vi "SetZForInte_modify_Bmode_temperature_SA Test.vi"(0 "TCP from Orchid in":refnum<k5>, 1 "timeout (ms)":dbl=40000.0 format="%.2f", 4 "RoiLaterMin":dbl format="%.2f", 5 "meas_temparature_Input":T2 {"scanRange" format="%.2f"; "temperatureC" format="%.2f"; "pulseVoltage" format="%.2f"; "roomTempC" format="%.2f"}, 9 "RoiLateralSpan":dbl format="%.2f", 11 "error in (no error)":errorcluster, 12 "meas_setting":T3={"measSetId"=6949, "measSetComments"="Orchid", "probeId"=141.0, "beamstyleIndex"=0, "txFrequencyHz"=3636400.0, "focusRangeCm"=8.0, "maxTxVoltageVolt"=100.0, "ceilTxVoltageVolt"=80.0, "profTxVoltageVolt"=62.0, "totalVoltagePt"=20, "numMeasVoltage"=12, "numTxElements"=118, "txpgWaveformStyle"=2, "numTxCycles"=4.0, "elevAperIndex"=0, "zStartDistCm"=1.5, "zMeasNum"=80, "IsTxAperModulationEn"=0, "DTxFreqIndex"=0, "VTxIndex"=0, "IsCPAEn"=0, "SysPulserSelA"=0, "TxPulseRleA"=""} {"zStartDistCm" format="%.2f"; "numTxCycles" format="%.1f"; "profTxVoltageVolt" format="%#_1g"; "ceilTxVoltageVolt" format="%.2f"; "maxTxVoltageVolt" format="%.2f"; "focusRangeCm" format="%.1f"; "txFrequencyHz" format="%.2f"}) -> (3 "Actual PRF":dbl, 6 "meas_temparature_Output":T1 {"scanRange" format="%.2f"; "txpgWaveformStyle" format="%.2f"; "temperatureC" format="%.2f"; "pulseVoltage" format="%.2f"; "roomTempC" format="%.2f"}, 10 "veri_P/F":bool, 15 "error out":errorcluster)   [LabVIEW 2016]
doc: "This VI sets the Z system transmit parameters for an intensity measurement, reads them back, and checks for errors. It first gets the initial center element delay (TxpgDelayAperA) and the system frequencies using tcpSysTxFreqFromZ.vi. It then sets the elevation aperture (using SetZElevAper.vi), channel modulation, wavestyle, frequency, focus, number of transmit elements, number of cycles, voltage, and voltage channel, in that order. It reads back the settings (using tcpReadIntenSettingsZ.vi) and checks for errors. The final trigger delay and change in delay, in microseconds, are calculated from the initial and final values of TxpgDelayAperA using:\ndelay(us) = (TxpgDelayAperA + 178.0) / 160"
uses:
  type def/measSetting.ctl
  GrobaLimitVoltage.vi
  TemperatureMeasure/Thermal_type.vi
panel:
  out "Receive array":string[](array[string])=["\r\n220 OK\r\nContainers within Hardware Control Layer\r\n\tHardwareModel\r\n\tHardwareControl\r\n\tHardwareAlgorithm\r\n\tSeq\r\n\tBeamforming\r\n\tDigitalReceiver\r\n\tEchoProcessor\r\n\tFlowProcessor\r\n\tHardwareScanConverter\r\n\tSip\r\n\tVideoInterface\r\n\tRtc\r\n\tCine\r\nScalar Parameters of Hardware Control Layer\r\nArray Parameters of Hardware Control Layer\r\ndebug\tDebug Functions\r\nquit\tExit DIOS\r\nback\tPrevious menu\r\nmain\tTop menu\r\nhelp\tAvailable commands\r\n\r\n", "\r\n220 OK\r\nContainers within Beamforming\r\n\tCommon\r\n\tBImage\r\n\tCbImage\r\n\tDImage\r\nScalar Parameters of Beamforming\r\nArray Parameters of Beamforming\r\ndebug\tDebug Functions\r\nquit\tExit DIOS\r\nback\tPrevious menu\r\nmain\tTop menu\r\nhelp\tAvailable commands\r\n\r\n", "\r\n220 OK\r\nContainers within Common\r\nScalar Parameters of Common\r\n\tBfPropagationVelCmPerSec\t154000\r\n\tDisUnit\t0.00385\r\n\tHwRcInterruptMask\t63\r\n\tHwRcTVP\t3\r\n\tHwRxAac0\t175\r\n\tHwRxAac1\t0\r\n\tHwRxbfBlankingWord\t0\r\n\tHwRxbfCmd1Word\t4232\r\n\tHwRxbfCmd2Word\t2\r\n\tHwRxbf0Cmd2Word\t3\r\n\tHwRxbfStartDelayWord\t10\r\n\tHwTiAttenuatorSelect\t0\r\n\tHwTiBitEn\t25088\r\n\tHwTiDacCtrl0\t255\r\n\tHwTiDacCtrl1\t2303\r\n\tHwTiDacCtrl2\t3327\r\n\tHwTiDacCtrl3\t511\r\n\tHwTiDacCtrl4\t2559\r\n\tHwTiDacCtrl5\t3583\r\n\tHwTiDacCtrl6\t767\r\n\tHwTiDacCtrl7\t2815\r\n\tHwTiDacCtrl8\t3839\r\n\tHwTiDacCtrl9\t2047\r\n\tHwTiDacCtrl10\t4095\r\n\tHwTiDigitalDriveCtrl\t0\r\n\tHwTiDigitalInterruptPolarity\t0\r\n\tHwTiDigitalReadCtrl\t0\r\n\tHwTiEchoBoosterCtrl\t0\r\n\tHwTiGlobalCtrl\t1\r\n\tHwTiHighVoltEn\t0\r\n\tHwTiInterruptClear\t65535\r\n\tHwTiInterruptMask\t32767\r\n\tHwTiMiscBitCtrl\t12\r\n\tHwTiProbeSelect\t2\r\n\tHwTiTXCLTransfer\t0\r\n\tHwTiVoltMultiplexer\t0\r\n\tHwTrGlobalCtrlAll\t1\r\n\tHwTrGlobalCtrl0All\t0\r\n\tHwTrDiagnosticCtrlAll\t0\r\n\tHwTrInterruptMaskAll\t1\r\n\tHwTrInterruptClearAll\t1\r\n\tHwTrRealTimeCtrlAll\t40\r\n\tHwTrTgcAacSignalCtrlAll\t0\r\n\tRxDelayRefx\t1\r\n\tRxDelayRefy\t-1\r\n\tTrPartNumber\t5928150\r\n\tBfPropagationVelFactor\t1\r\n\tDigitizingRateHz\t4e+007\r\n\tHwRxBfVectorLengthWord\t0\r\n\tIsRxVectorLengthEn\t1\r\n\tNumChannels\t192\r\n\tProbeBandwidthHz\t3.6e+006\r\n\tProbeId\t171\r\n\tProbeNumElem\t192\r\n\tProbeNumRows\t1\r\n\tProbePitchCm\t0.02\r\n\tProbeRadiusElectricalCm\t0\r\n\tProbeType\t0\r\n\tPropagationVelCmPerSec\t154000\r\n\tRxApod2dEn\t0\r\n\tRxbfAdcDelayClocks\t10\r\n\tRxbfGainShift\t0\r\n\tRxDelayYOffsetSysClk4\t0\r\n\tTxPulserMaxVolt\t50\r\nArray Parameters of Common\r\n\tHwRxbf0AdGainA\tsize=64\r\n\tHwRxbf1AdGainA\tsize=64\r\n\tHwRxbf2AdGainA\tsize=64\r\n\tHwRxbf3AdGainA\tsize=64\r\n\tHwRxbf4AdGainA\tsize=64\r\n\tHwRxbf5AdGainA\tsize=64\r\n\tHwRxbf6AdGainA\tsize=64\r\n\tHwRxbf7AdGainA\tsize=64\r\n\tHwRxbf8AdGainA\tsize=64\r\n\tHwRxbf9AdGainA\tsize=64\r\n\tHwRxbf10AdGainA\tsize=64\r\n\tHwRxbf11AdGainA\tsize=64\r\n\tHwRxAdOffsetCalA\tsize=192\r\n\tHwRxApodFilterRamA\tsize=512\r\n\tHwRxbf0DelayCalA\tsize=64\r\n\tHwRxbf1DelayCalA\tsize=64\r\n\tHwRxbf2DelayCalA\tsize=64\r\n\tHwRxbf3DelayCalA\tsize=64\r\n\tHwRxbf4DelayCalA\tsize=64\r\n\tHwRxbf5DelayCalA\tsize=64\r\n\tHwRxbf6DelayCalA\tsize=64\r\n\tHwRxbf7DelayCalA\tsize=64\r\n\tHwRxbf8DelayCalA\tsize=64\r\n\tHwRxbf9DelayCalA\tsize=64\r\n\tHwRxbf10DelayCalA\tsize=64\r\n\tHwRxbf11DelayCalA\tsize=64\r\n\tHwRxbf0DxA\tsize=64\r\n\tHwRxbf1DxA\tsize=64\r\n\tHwRxbf2DxA\tsize=64\r\n\tHwRxbf3DxA\tsize=64\r\n\tHwRxbf4DxA\tsize=64\r\n\tHwRxbf5DxA\tsize=64\r\n\tHwRxbf6DxA\tsize=64\r\n\tHwRxbf7DxA\tsize=64\r\n\tHwRxbf8DxA\tsize=64\r\n\tHwRxbf9DxA\tsize=64\r\n\tHwRxbf10DxA\tsize=64\r\n\tHwRxbf11DxA\tsize=64\r\n\tHwRxbf0DyA\tsize=64\r\n\tHwRxbf1DyA\tsize=64\r\n\tHwRxbf2DyA\tsize=64\r\n\tHwRxbf3DyA\tsize=64\r\n\tHwRxbf4DyA\tsize=64\r\n\tHwRxbf5DyA\tsize=64\r\n\tHwRxbf6DyA\tsize=64\r\n\tHwRxbf7DyA\tsize=64\r\n\tHwRxbf8DyA\tsize=64\r\n\tHwRxbf9DyA\tsize=64\r\n\tHwRxbf10DyA\tsize=64\r\n\tHwRxbf11DyA\tsize=64\r\n\tHwRxbf0DzA\tsize=128\r\n\tHwRxbf1DzA\tsize=128\r\n\tHwRxbf2DzA\tsize=128\r\n\tHwRxbf3DzA\tsize=128\r\n\tHwRxbf4DzA\tsize=128\r\n\tHwRxbf5DzA\tsize=128\r\n\tHwRxbf6DzA\tsize=128\r\n\tHwRxbf7DzA\tsize=128\r\n\tHwRxbf8DzA\tsize=128\r\n\tHwRxbf9DzA\tsize=128\r\n\tHwRxbf10DzA\tsize=128\r\n\tHwRxbf11DzA\tsize=128\r\n\tHwRxbf0PosInApodWinA\tsize=64\r\n\tHwRxbf1PosInApodWinA\tsize=64\r\n\tHwRxbf2PosInApodWinA\tsize=64\r\n\tHwRxbf3PosInApodWinA\tsize=64\r\n\tHwRxbf4PosInApodWinA\tsize=64\r\n\tHwRxbf5PosInApodWinA\tsize=64\r\n\tHwRxbf6PosInApodWinA\tsize=64\r\n\tHwRxbf7PosInApodWinA\tsize=64\r\n\tHwRxbf8PosInApodWinA\tsize=64\r\n\tHwRxbf9PosInApodWinA\tsize=64\r\n\tHwRxbf10PosInApodWinA\tsize=64\r\n\tHwRxbf11PosInApodWinA\tsize=64\r\n\tHwRxMuxSelectLutA\tsize=512\r\n\tHwRxRamOffsetA\tsize=12\r\n\tHwTxDacA\tsize=2\r\n\tHwTxpgDelayAperA\tsize=393216\r\n\tNumBitsPerCycleA\tsize=49\r\n\tNumCyclesPerPassA\tsize=49\r\n\tNumWordsPerPassA\tsize=49\r\n\tRxAdGainA\tsize=256\r\n\tRxDelayCalA\tsize=768\r\n\tRxDxA\tsize=256\r\n\tRxDyA\tsize=256\r\n\tRxDzA\tsize=256\r\n\tRxMuxSelectLutPtrA\tsize=512\r\n\tRxPosInApodWinA\tsize=768\r\n\tTxDelayCalA\tsize=192\r\n\tTxpgWaveformHoutA\tsize=15680\r\n\tTxpgWaveformLoutA\tsize=15680\r\n\tYIndexTableA\tsize=256\r\n\tZIndexTableA\tsize=256\r\n\tInsertedProbeIdA\tsize=6\r\n\tPulseVoltageA\tsize=2\r\n\tRxApodFactorA\tsize=4\r\n\tRxApodSelA\tsize=4\r\n\tSysTxFreqHzA\tsize=49\r\ndebug\tDebug Functions\r\nquit\tExit DIOS\r\nback\tPrevious menu\r\nmain\tTop menu\r\nhelp\tAvailable commands\r\n\r\n", "220 OK\r\n", "250 20\r\n"]
  out "error out 2":errorcluster
  out "Pass_count":i16
  out "All_param_veri":bool[](array[boolean])
  in  "volt channel":i8
  # "Program constants"
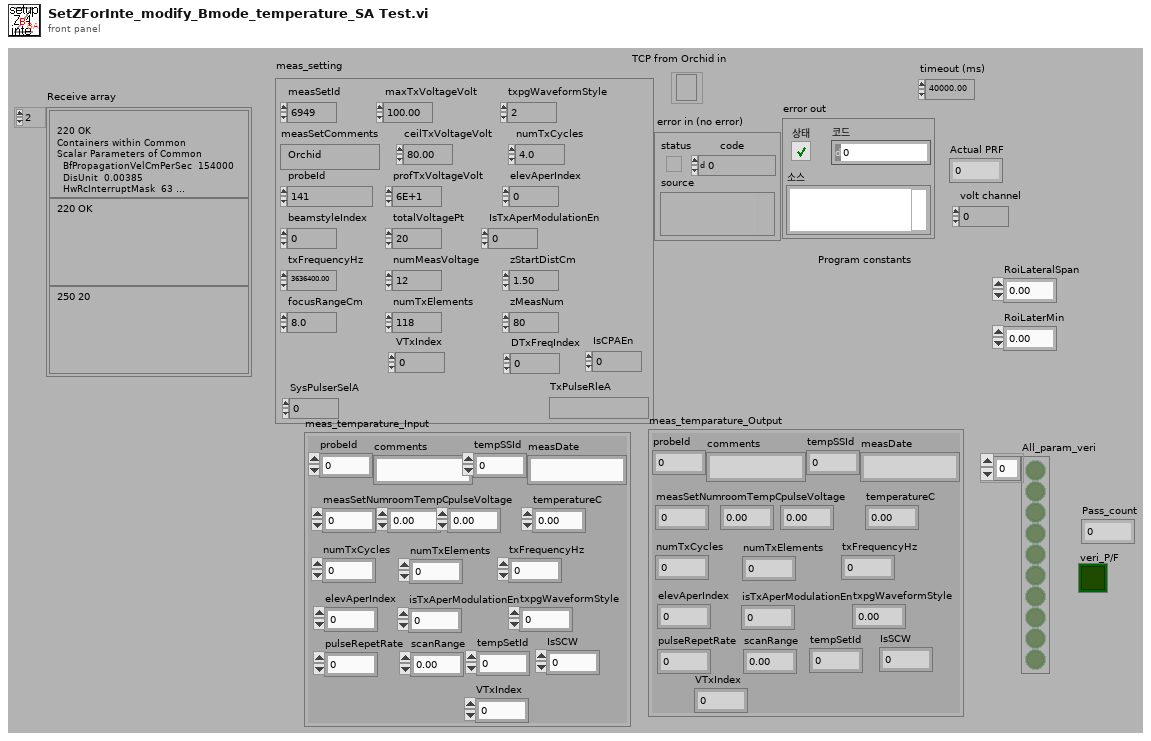
[diagram p1: front panel]
types:
  T1 = cluster{"probeId":sgl, "comments":string, "tempSSId":i16, "measDate":string, "measSetNum":i16, "roomTempC":sgl, "pulseVoltage":dbl, "temperatureC":ext, "numTxCycles":dbl, "numTxElements":i16, "txFrequencyHz":i32, "elevAperIndex":i16, "isTxAperModulationEn":i16, "txpgWaveformStyle":sgl, "pulseRepetRate":i32, "scanRange":dbl, "tempSetId":i16, "IsSCW":i16, "VTxIndex":i32}
  T2 = cluster{"probeId":sgl, "comments":string, "tempSSId":i16, "measDate":string, "measSetNum":i16, "roomTempC":sgl, "pulseVoltage":dbl, "temperatureC":ext, "numTxCycles":dbl, "numTxElements":i16, "txFrequencyHz":i32, "elevAperIndex":i16, "isTxAperModulationEn":i16, "txpgWaveformStyle":i16, "pulseRepetRate":dbl, "scanRange":dbl, "tempSetId":i16, "IsSCW":i16, "VTxIndex":i16}
  T3 = typedef "measSetting.ctl" = cluster{"measSetId":i32, "measSetComments":string, "probeId":sgl, "beamstyleIndex":i16, "txFrequencyHz":sgl, "focusRangeCm":sgl, "maxTxVoltageVolt":sgl, "ceilTxVoltageVolt":sgl, "profTxVoltageVolt":dbl, "totalVoltagePt":i8, "numMeasVoltage":i8, "numTxElements":i16, "txpgWaveformStyle":i8, "numTxCycles":sgl, "elevAperIndex":i8, "zStartDistCm":sgl, "zMeasNum":i8, "IsTxAperModulationEn":i8, "DTxFreqIndex":i16, "VTxIndex":i8, "IsCPAEn":i16, "SysPulserSelA":i16, "TxPulseRleA":string}
  T4 = cluster{"numTxCycles":dbl, "numTxElements":i16, "txFrequencyIndex":i32, "isTxAperModulationEn":i16, "txpgWaveformStyle":i16, "pulseRepetRate":dbl, "RoiLateralSpan":dbl, "RoiLateralMin":dbl}
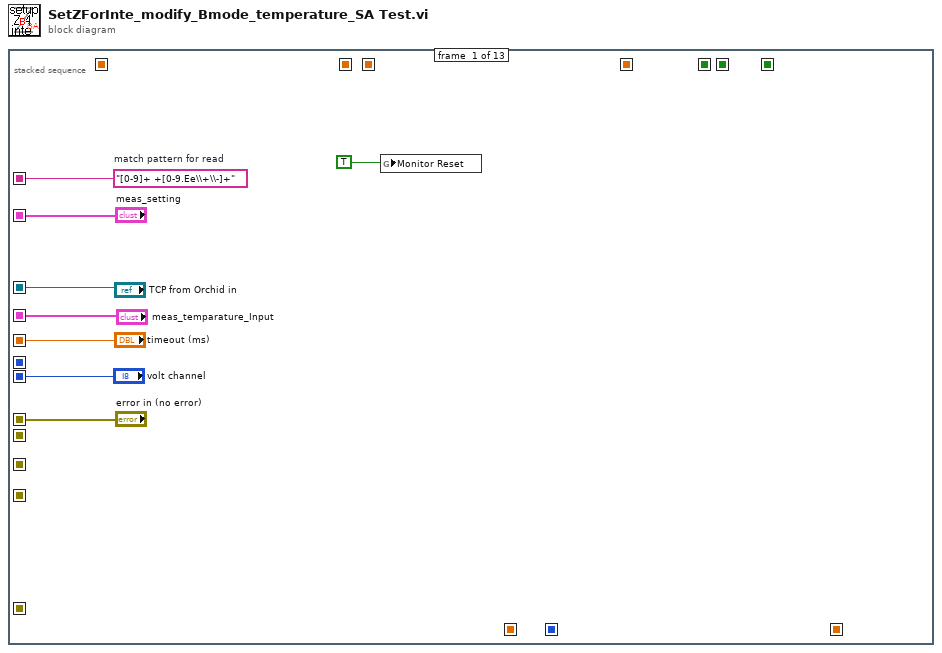
[diagram p0: block diagram]
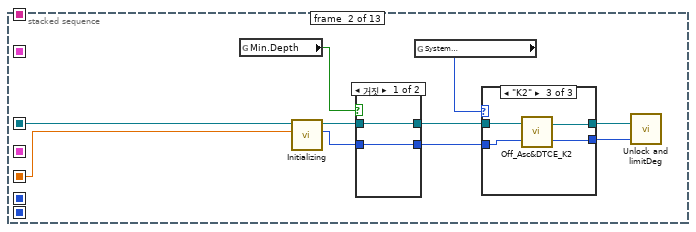
[diagram p2: hidden frame]
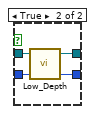
[diagram p3: hidden frame]
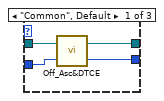
[diagram p4: hidden frame]
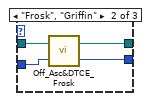
[diagram p5: hidden frame]
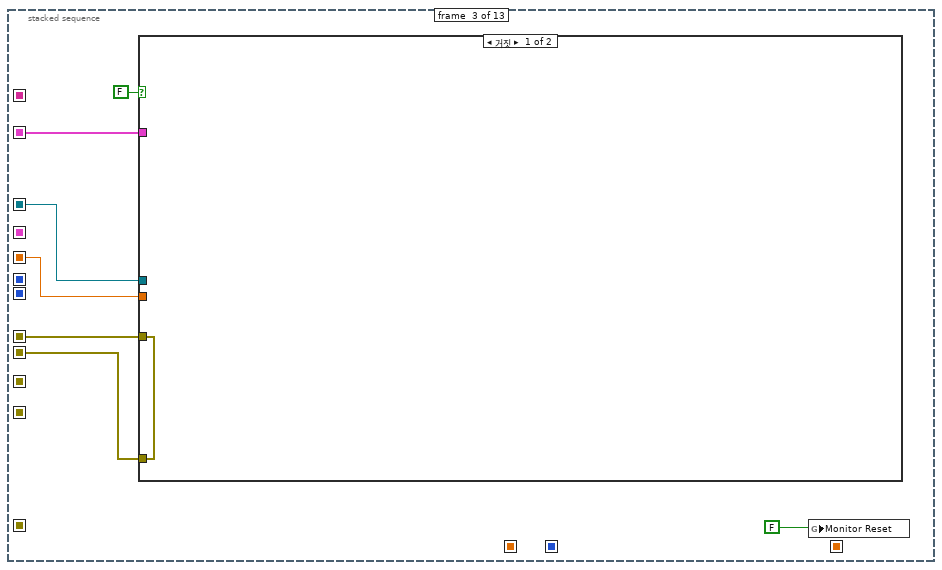
[diagram p6: hidden frame]
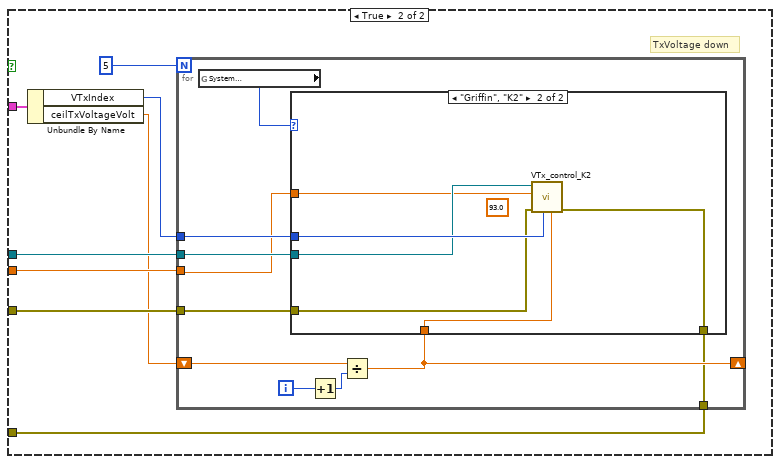
[diagram p7: hidden frame]
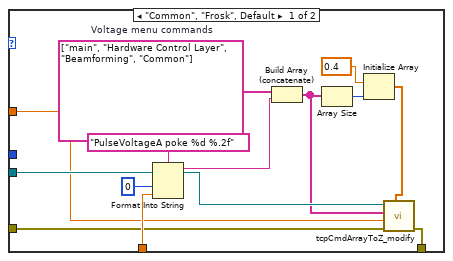
[diagram p8: hidden frame]
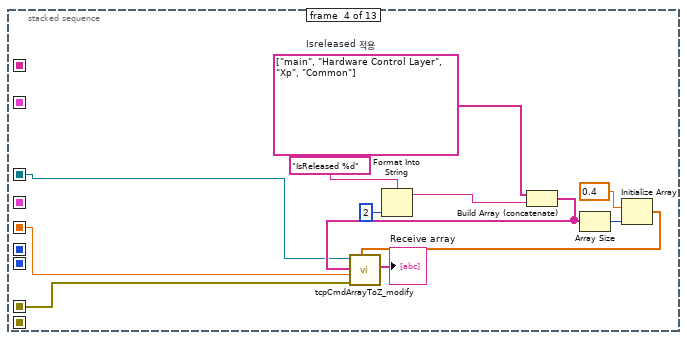
[diagram p9: hidden frame]
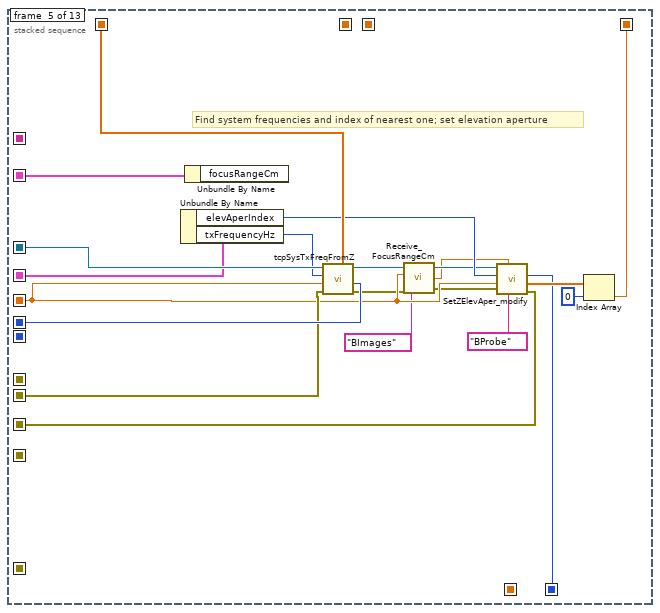
[diagram p10: hidden frame]
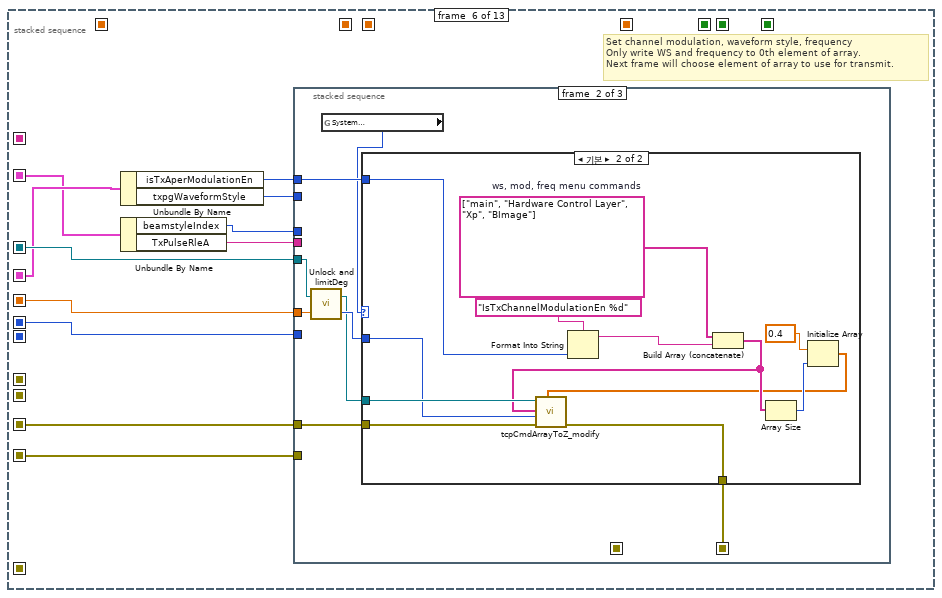
[diagram p11: hidden frame]
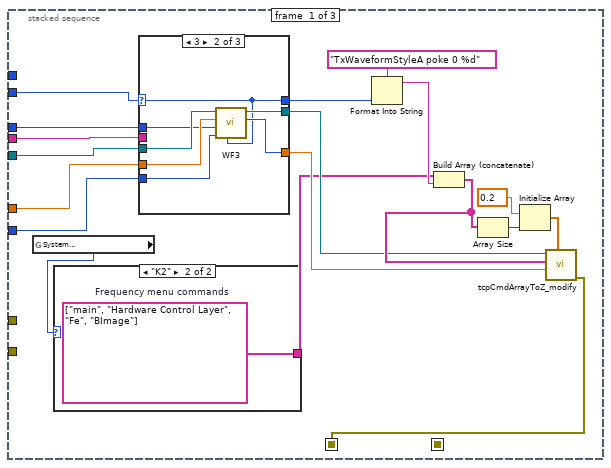
[diagram p12: hidden frame]
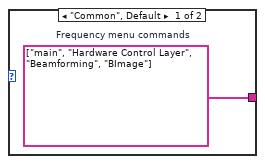
[diagram p13: hidden frame]
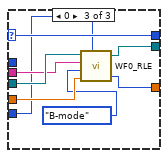
[diagram p15: hidden frame]
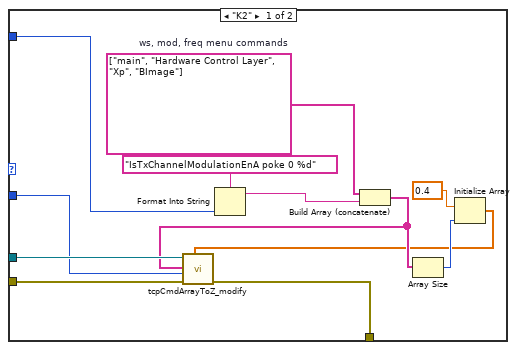
[diagram p16: hidden frame]
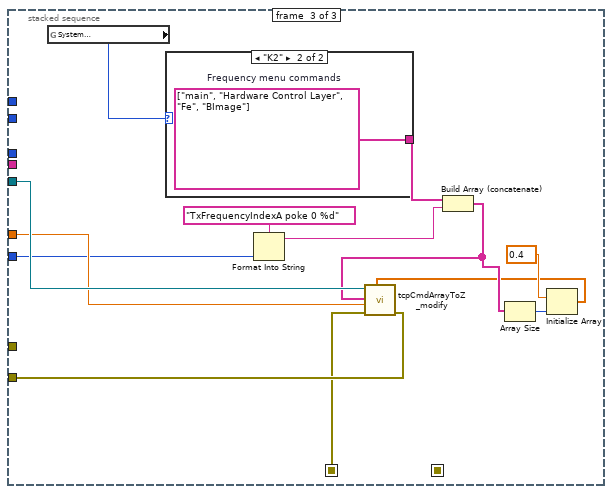
[diagram p17: hidden frame]
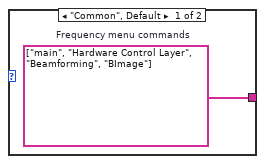
[diagram p18: hidden frame]
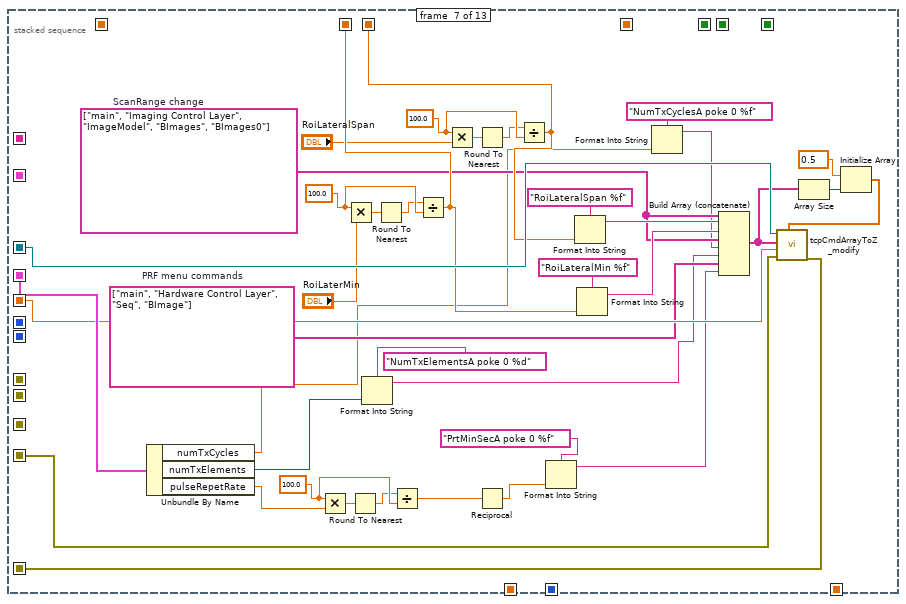
[diagram p19: hidden frame]
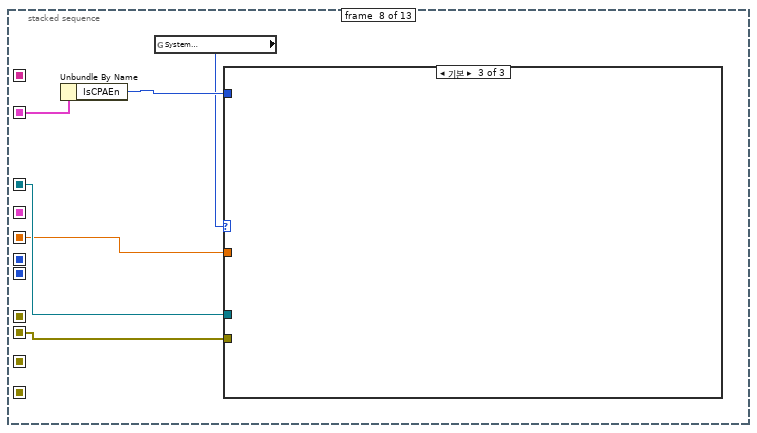
[diagram p20: hidden frame]
diagram:
  n1 = stacked-sequence {
    seq-local: ["meas_temparature_Input" _ _ _ _ _ _ _ _ _ _ _ _] -> [_ _ _ _ w113 w120 w249 _ _ w336 w359 _ _]
    seq-local: ["TCP from Orchid in" _ _ _ _ _ _ _ _ _ _ _ _] -> [_ w18 w41 w84 w114 w125 w247 w255 w281 w335 w352 w400 w414]
    seq-local: ["timeout (ms)" _ _ _ _ _ _ _ _ _ _ _ _] -> [_ w17 w40 w82 w97 w124 w246 w254 w280 w334 w351 w399 w413]
    seq-local: [_ _ _ _ w112 _ _ _ _ _ _ _ _] -> [_ _ _ _ _ w121 _ _ _ w340 _ _ _]
    seq-local: [_ _ _ _ w104 _ _ _ _ _ _ _ _] -> [_ _ _ _ _ w122 _ _ _ _ _ _ _]
    seq-local: [_ _ _ _ w111 _ _ _ _ _ _ _ _] -> [_ _ _ _ _ _ _ _ _ _ _ _ _]
    seq-local: ["volt channel" _ _ _ _ _ _ _ _ _ _ _ _] -> [_ _ _ _ _ _ _ _ _ _ _ _ _]
    seq-local: ["error in (no error)" _ _ _ _ _ _ _ _ _ _ _ _] -> [_ _ w39 w83 _ _ _ _ _ _ _ _ _]
    seq-local: [w5 _ _ _ _ _ _ _ _ _ _ _ _] -> [_ _ _ _ _ _ _ _ _ _ _ _ _]
    seq-local: [_ _ w38 _ _ _ _ _ _ _ _ _ _] -> [_ _ _ _ w109 _ _ w252 w279 _ _ _ _]
    seq-local: [_ _ _ _ _ w123 _ _ _ _ _ _ _] -> [_ _ _ _ _ _ w248 _ _ _ _ _ _]
    seq-local: [_ _ _ _ _ _ w245 _ _ _ _ _ _] -> [_ _ _ _ _ _ _ _ _ _ w349 _ _]
    seq-local: ["meas_setting" _ _ _ _ _ _ _ _ _ _ _ _] -> [_ _ w43 _ w102 w119 _ w253 _ w316 w354 _ _]
    seq-local: [_ _ _ _ _ _ w243 _ _ _ _ _ _] -> [_ _ _ _ _ _ _ _ _ w338 _ _ _]
    seq-local: [_ _ _ _ _ _ w244 _ _ _ _ _ _] -> [_ _ _ _ _ _ _ _ _ w339 _ _ _]
    seq-local: [_ _ _ _ _ _ _ _ _ _ w348 _ _] -> [_ _ _ _ _ _ _ _ _ _ _ _ _]
    seq-local: [_ _ _ _ _ _ _ _ _ w337 _ _ _] -> [_ _ _ _ _ _ _ _ _ _ _ w398 _]
    seq-local: [_ _ _ _ _ _ _ _ _ _ w346 _ _] -> [_ _ _ _ _ _ _ _ _ _ _ w397 _]
    seq-local: [_ _ _ _ w103 _ _ _ _ _ _ _ _] -> [_ _ _ _ _ _ _ _ _ _ _ _ _]
    seq-local: [_ _ _ _ w101 _ _ _ _ _ _ _ _] -> [_ _ _ _ _ _ _ _ _ _ _ _ _]
    seq-local: [_ _ _ _ _ _ _ _ _ w312 _ _ _] -> [_ _ _ _ _ _ _ _ _ _ _ w395 _]
    seq-local: [_ _ _ _ _ _ _ _ w278 _ _ _ _] -> [_ _ _ _ _ _ _ _ _ w310 _ _ _]
    frame #0 {
      w5 = "[0-9]+ +[0-9.Ee\\+\\-]+"  # match pattern for read
      n2 = global write "GrobaLimitVoltage.vi" "Monitor Reset"(TRUE) -> ()
    }
    frame #1 {
      n3 = global read "Thermal_type.vi" "Min.Depth"() -> (w9:bool)
      n4 = call "Initializing.vi"("Timeout (ms)"=w17, "connection ID in"=w18) -> ("Timeout (ms) 2"=w12:i32, "connection ID in 2"=w13:refnum<k5>)  [unwired: 8 in]
      n5 = case shown="거짓" w9 {
        tunnel: w13 -> [w20 w24]
        tunnel: w12 -> [w19 w23]
        tunnel: [w20 w22] -> w11
        tunnel: [w19 w21] -> w10
        frame False {
        }
        frame True {
          n6 = call "Low_Depth.vi"("Timeout (ms)"=w23, "connection ID in"=w24) -> ("Timeout (ms) 2"=w21:i32, "connection ID out"=w22:refnum<k5>)  [unwired: 2 in]
        }
      }
      n7 = global read "Thermal_type.vi" "System \nSelection"() -> (w16:enum32{"Common", "Frosk", "Griffin", "K2"})
      n8 = case shown="\"K2\"" w16 {
        tunnel: [w28 w32 w34] -> w15
        tunnel: [w27 w31 w33] -> w14
        tunnel: w11 -> [w26 w30 w36]
        tunnel: w10 -> [w25 w29 w35]
        frame "Common", Default {
          n9 = call "Off_Asc&DTCE.vi"("Timeout (ms)"=w25, "connection ID in"=w26) -> ("Timeout (ms) 2"=w27:i32, "connection ID out"=w28:refnum<k5>)
        }
        frame "Frosk", "Griffin" {
          n10 = call "Off_Asc&DTCE_Frosk.vi"("Timeout (ms)"=w29, "connection ID in"=w30) -> ("Timeout (ms) 2"=w31:i32, "connection ID out"=w32:refnum<k5>)
        }
        frame "K2" {
          n11 = call "Off_Asc&DTCE_K2.vi"("Timeout (ms)"=w35, "connection ID in"=w36) -> ("Timeout (ms) 2"=w33:i32, "connection ID out"=w34:refnum<k5>)
        }
      }
      n12 = call "Unlock and limitDeg.vi"("Timeout (ms)"=w14, "connection ID in"=w15) -> ()  [unwired: 2 out]
    }
    frame #2 {
      n13 = case shown="거짓" FALSE {
        tunnel: w43 -> [_ w52]
        tunnel: w41 -> [_ w49]
        tunnel: w40 -> [_ w48]
        tunnel: w39 -> [w44 w47]
        tunnel: [w44 w46] -> w38
        frame False {
        }
        frame True {
          # "TxVoltage down"
          n14 = Unbundle By Name(w52) -> ("VTxIndex"=w50:i8, "ceilTxVoltageVolt"=w45:sgl)
          n15 = for {
            N: 5 -> [_]
            tunnel: w49 -> [w62]
            shift-right: [w56] -> _
            shift-left: w45 -> [w58]
            tunnel: w50 -> [w61]
            tunnel: [w55] -> w46
            tunnel: w48 -> [w54]
            tunnel: w47 -> [w53]
            i -> [w57]
            n16 = global read "Thermal_type.vi" "System \nSelection"() -> (w60:enum32{"Common", "Frosk", "Griffin", "K2"})
            n17 = Increment(x=w57) -> (x+1=w59:i32)
            n18 = Divide(x=w58, y=w59) -> (x/y=w56:sgl)
            n19 = case shown="\"Griffin\", \"K2\"" w60 {
              tunnel: w62 -> [w75 w80]
              tunnel: w61 -> [_ w81]
              tunnel: w56 -> [w66 w79]
              tunnel: [w65 w78] -> w55
              tunnel: w54 -> [w63 w77]
              tunnel: w53 -> [w64 w76]
              frame "Common", "Frosk", Default {
                w73 = string[] ["main", "Hardware Control Layer", "Beamforming", "Common"]  # Voltage menu commands
                n20 = Format Into String(format string="PulseVoltageA poke %d %.2f" ("Format String"), i8 0 ("입력 1"), w66) -> (resulting string=w72:string)  [unwired: 2 in, 1 out]
                n21 = Build Array (concatenate)(w73, w72) -> (w68:string[])
                n22 = Array Size(array=w68) -> (size(s)=w71:i32)
                n23 = Initialize Array(0.4 ("element"), w71) -> (w69:dbl[])
                n24 = call "tcpCmdArrayToZ_modify.vi"("Delay (sec)"=w69, "error in (no error)"=w64, "Timeout (ms)"=w63, "Command array"=w68, "connection ID in"=w75) -> ("error out"=w65:errorcluster)  [unwired: 2 in, 4 out]
              }
              frame "Griffin", "K2" {
                (unwired) 93.0 ("VTx1_voltage")
                n25 = call "VTx_control_K2.vi"("VTx_Voltage"=w79, "VTxIndex_In"=w81, "error in (no error)"=w76, "Timeout (ms)"=w77, "connection ID in"=w80) -> ("error out"=w78:errorcluster)  [unwired: 5 in, 1 out]
              }
            }
          }
        }
      }
      n26 = global write "GrobaLimitVoltage.vi" "Monitor Reset"(FALSE) -> ()
    }
    frame #3 {
      w87 = string[] ["main", "Hardware Control Layer", "Xp", "Common"]  # Isreleased 적용
      n27 = Format Into String(format string="IsReleased %d" ("Format String"), i16 2 ("입력 1")) -> (resulting string=w92:string)  [unwired: 2 in, 1 out]
      n28 = Build Array (concatenate)(w87, w92) -> (w89:string[])
      n29 = Array Size(array=w89) -> (size(s)=w91:i32)
      n30 = Initialize Array(0.4 ("element"), w91) -> (w88:dbl[])
      n31 = call "tcpCmdArrayToZ_modify.vi"("Delay (sec)"=w88, "error in (no error)"=w83, "Timeout (ms)"=w82, "Command array"=w89, "connection ID in"=w84) -> ("Receive array"=→"Receive array":string[])  [unwired: 2 in, 4 out]
    }
    frame #4 {
      # "Find system frequencies and index of nearest one; set elevation aperture"
      n32 = Unbundle By Name(w113) -> ("elevAperIndex"=w105:i16, "txFrequencyHz"=w110:i32)
      n33 = Unbundle By Name(w102) -> ()  [unwired: 1 out]
      n34 = call "tcpSysTxFreqFromZ.vi"("error in (no error)"=w109, "timeout (ms)"=w97, "txFrequencyHz in"=w110, "connection ID in"=w114) -> ("error out"=w95:errorcluster, "TxFreqIndex"=w112:i8, "connection ID out"=w100:refnum<k5>, "SysTxFreqHzA"=w111:sgl[])  [unwired: 3 in, 1 out]
      n35 = call "Receive_FocusRangeCm.vi"("error in (no error)"=w95, "Image mode"="BImages", "Timeout (ms)"=w97, "connection ID in"=w100) -> ("error out"=w94:errorcluster, "FocusRangeCm"=w98:dbl, "connection ID out"=w99:refnum<k5>)
      n36 = call "SetZElevAper_modify.vi"("Mode"="BProbe", "focusRangeCm"=w98, "error in (no error)"=w94, "timeout (ms)"=w97, "elevAperIndex"=w105, "connection ID in"=w99) -> ("error out"=w104:errorcluster, "SwitchDepth"=w107:sgl[], "probeNumElevAper"=w103:i32)  [unwired: 2 in, 1 out]
      n37 = Index Array(array=w107, index=0 ("인덱스")) -> (element=w101:sgl)
    }
    frame #5 {
      # "Set channel modulation, waveform style, frequency\nOnly write WS and frequency to 0th element of array.\nNext frame will choose element of array to use for transmit."
      n38 = Unbundle By Name(w120) -> ("isTxAperModulationEn"=w118:i16, "txpgWaveformStyle"=w117:i16)
      n39 = Unbundle By Name(w119) -> ("beamstyleIndex"=w116:i16, "TxPulseRleA"=w115:string)
      n40 = stacked-sequence {
        seq-local: [w128 _ _] -> [_ _ w196]
        seq-local: [_ w169 _] -> [_ _ _]
        tunnel: w125 -> [w138 w165 w208]
        tunnel: w124 -> [w137 w164 w207]
        tunnel: [_ _ w206] -> w123
        tunnel: w122 -> [_ w170 _]
        tunnel: w121 -> [w136 _ w204]
        tunnel: w118 -> [_ w171 _]
        tunnel: w117 -> [w127 _ _]
        tunnel: w116 -> [w135 _ _]
        tunnel: w115 -> [w126 _ _]
        frame #0 {
          n41 = global read "Thermal_type.vi" "System \nSelection"() -> (w129:enum32{"Common", "Frosk", "Griffin", "K2"})
          n42 = case shown="\"K2\"" w129 {
            tunnel: [w144 w145] -> w130
            frame "Common", Default {
              w144 = string[] ["main", "Hardware Control Layer", "Beamforming", "BImage"]  # Frequency menu commands
            }
            frame "K2" {
              w145 = string[] ["main", "Hardware Control Layer", "Fe", "BImage"]  # Frequency menu commands
            }
          }
          n43 = case shown="3" w127 {
            selector: w127 -> [w146 w149 w160]
            tunnel: w138 -> [w148 w155 w163]
            tunnel: [w148 w154 w159] -> w133
            tunnel: [w147 w153 w158] -> w132
            tunnel: w137 -> [w147 w152 w161]
            tunnel: w135 -> [_ w151 _]
            tunnel: w136 -> [_ w150 w156]
            tunnel: [w146 w149 w160] -> w134
            tunnel: w126 -> [_ _ w162]
            frame Default {
            }
            frame 3 {
              n44 = call "WF3.vi"("TxWaveformStyle"=w149, "TxFreqIndex"=w150, "BeamStyleIndex"=w151, "Timeout (ms)"=w152, "connection ID in"=w155) -> ("Timeout (ms) out"=w153:i32, "connection ID out"=w154:refnum<k5>)  [unwired: 5 in]
            }
            frame 0 {
              n45 = call "WF0_RLE.vi"("connection ID in"=w163, "TxPulseRleA"=w162, "Mode control"=enum32{"D-mode", "B-mode"}."B-mode", "Timeout (ms)"=w161, "TxFrequencyIndex"=w156) -> ("connection ID out"=w159:refnum<k5>, "Timeout (ms) out"=w158:i32)  [unwired: 1 in]
            }
          }
          n46 = Format Into String(format string="TxWaveformStyleA poke 0 %d" ("Format String"), w134) -> (resulting string=w131:string)  [unwired: 2 in, 1 out]
          n47 = Build Array (concatenate)(w130, w131) -> (w140:string[])
          n48 = Array Size(array=w140) -> (size(s)=w142:i32)
          n49 = Initialize Array(0.2 ("element"), w142) -> (w139:dbl[])
          n50 = call "tcpCmdArrayToZ_modify.vi"("Delay (sec)"=w139, "Timeout (ms)"=w132, "Command array"=w140, "connection ID in"=w133) -> ("error out"=w128:errorcluster)  [unwired: 3 in, 4 out]
        }
        frame #1 {
          n51 = call "Unlock and limitDeg.vi"("Timeout (ms)"=w164, "connection ID in"=w165) -> ("Timeout (ms) 2"=w167:i32, "connection ID out"=w166:refnum<k5>)
          n52 = global read "Thermal_type.vi" "System \nSelection"() -> (w168:enum32{"Common", "Frosk", "Griffin", "K2"})
          n53 = case shown="기본" w168 {
            tunnel: w166 -> [w183 w195]
            tunnel: w167 -> [w182 w194]
            tunnel: w171 -> [w175 w187]
            tunnel: w170 -> [w173 w185]
            tunnel: [w172 w184] -> w169
            frame "K2" {
              w174 = string[] ["main", "Hardware Control Layer", "Xp", "BImage"]  # ws, mod, freq menu commands
              n54 = Format Into String(format string="IsTxChannelModulationEnA poke 0 %d" ("Format String"), w175) -> (resulting string=w180:string)  [unwired: 2 in, 1 out]
              n55 = Build Array (concatenate)(w174, w180) -> (w177:string[])
              n56 = Array Size(array=w177) -> (size(s)=w179:i32)
              n57 = Initialize Array(0.4 ("element"), w179) -> (w176:dbl[])
              n58 = call "tcpCmdArrayToZ_modify.vi"("Delay (sec)"=w176, "error in (no error)"=w173, "Timeout (ms)"=w182, "Command array"=w177, "connection ID in"=w183) -> ("error out"=w172:errorcluster)  [unwired: 2 in, 4 out]
            }
            frame Default {
              w186 = string[] ["main", "Hardware Control Layer", "Xp", "BImage"]  # ws, mod, freq menu commands
              n59 = Format Into String(format string="IsTxChannelModulationEn %d" ("Format String"), w187) -> (resulting string=w192:string)  [unwired: 2 in, 1 out]
              n60 = Build Array (concatenate)(w186, w192) -> (w189:string[])
              n61 = Array Size(array=w189) -> (size(s)=w191:i32)
              n62 = Initialize Array(0.4 ("element"), w191) -> (w188:dbl[])
              n63 = call "tcpCmdArrayToZ_modify.vi"("Delay (sec)"=w188, "error in (no error)"=w185, "Timeout (ms)"=w194, "Command array"=w189, "connection ID in"=w195) -> ("error out"=w184:errorcluster)  [unwired: 2 in, 4 out]
            }
          }
        }
        frame #2 {
          n64 = global read "Thermal_type.vi" "System \nSelection"() -> (w198:enum32{"Common", "Frosk", "Griffin", "K2"})
          n65 = case shown="\"K2\"" w198 {
            tunnel: [w209 w210] -> w197
            frame "Common", Default {
              w209 = string[] ["main", "Hardware Control Layer", "Beamforming", "BImage"]  # Frequency menu commands
            }
            frame "K2" {
              w210 = string[] ["main", "Hardware Control Layer", "Fe", "BImage"]  # Frequency menu commands
            }
          }
          n66 = Format Into String(format string="TxFrequencyIndexA poke 0 %d" ("Format String"), w204) -> (resulting string=w203:string)  [unwired: 2 in, 1 out]
          n67 = Build Array (concatenate)(w197, w203) -> (w200:string[])
          n68 = Array Size(array=w200) -> (size(s)=w202:i32)
          n69 = Initialize Array(0.4 ("element"), w202) -> (w199:dbl[])
          n70 = call "tcpCmdArrayToZ_modify.vi"("Delay (sec)"=w199, "error in (no error)"=w196, "Timeout (ms)"=w207, "Command array"=w200, "connection ID in"=w208) -> ("error out"=w206:errorcluster)  [unwired: 2 in, 4 out]
        }
      }
    }
    frame #6 {
      w219 = 100.0
      w223 = 100.0
      w227 = 100.0
      w232 = string[] ["main", "Imaging Control Layer", "ImageModel", "BImages", "BImages0"]  # ScanRange change
      w234 = string[] ["main", "Hardware Control Layer", "Seq", "BImage"]  # PRF menu commands
      n71 = Unbundle By Name(w249) -> ("numTxCycles"=w229:dbl, "numTxElements"=w236:i16, "pulseRepetRate"=w217:dbl)
      n72 = Multiply(x=w219, y=w217) -> (x*y=w220:dbl)
      n73 = Multiply(x=w223, y="RoiLaterMin") -> (x*y=w224:dbl)
      n74 = Round To Nearest(number=w220) -> (nearest integer value=w218:dbl)
      n75 = Format Into String(format string="NumTxElementsA poke 0 %d" ("Format String"), w236) -> (resulting string=w233:string)  [unwired: 2 in, 1 out]
      n76 = Round To Nearest(number=w224) -> (nearest integer value=w222:dbl)
      n77 = Divide(x=w218, y=w219) -> (x/y=w212:dbl)
      n78 = Divide(x=w222, y=w223) -> (x/y=w243:dbl)
      n79 = Multiply(x=w227, y="RoiLateralSpan") -> (x*y=w228:dbl)
      n80 = Round To Nearest(number=w228) -> (nearest integer value=w226:dbl)
      n81 = Reciprocal(x=w212) -> (1/x=w211:dbl)
      n82 = Divide(x=w226, y=w227) -> (x/y=w244:dbl)
      n83 = Format Into String(format string="PrtMinSecA poke 0 %f", w211) -> (resulting string=w235:string)  [unwired: 2 in, 1 out]
      n84 = Format Into String(format string="RoiLateralSpan %f", w244) -> (resulting string=w239:string)  [unwired: 2 in, 1 out]
      n85 = Format Into String(format string="RoiLateralMin %f", w243) -> (resulting string=w238:string)  [unwired: 2 in, 1 out]
      n86 = Format Into String(format string="NumTxCyclesA poke 0 %f" ("Format String"), w229) -> (resulting string=w230:string)  [unwired: 2 in, 1 out]
      n87 = Build Array (concatenate)(w232, w239, w238, w232, w230, w233, w234, w235) -> (w214:string[])
      n88 = Array Size(array=w214) -> (size(s)=w216:i32)
      n89 = Initialize Array(0.5 ("element"), w216) -> (w213:dbl[])
      n90 = call "tcpCmdArrayToZ_modify.vi"("Delay (sec)"=w213, "error in (no error)"=w248, "Timeout (ms)"=w246, "Command array"=w214, "connection ID in"=w247) -> ("error out"=w245:errorcluster)  [unwired: 2 in, 4 out]
    }
    frame #7 {
      n91 = Unbundle By Name(w253) -> ("IsCPAEn"=w251:i16)
      n92 = global read "Thermal_type.vi" "System \nSelection"() -> (w250:enum32{"Common", "Frosk", "Griffin", "K2"})
      n93 = case shown="기본" w250 {
        tunnel: w255 -> [w266 w277 _]
        tunnel: w254 -> [w265 w276 _]
        tunnel: w251 -> [w258 w269 _]
        tunnel: w252 -> [w256 w267 _]
        frame "K2" {
          w257 = string[] ["main", "Hardware Control Layer", "Fe", "BImage"]  # ws, mod, freq menu commands
          n94 = Format Into String(format string="IsCPAEn %d" ("Format String"), w258) -> (resulting string=w263:string)  [unwired: 2 in, 1 out]
          n95 = Build Array (concatenate)(w257, w263) -> (w260:string[])
          n96 = Array Size(array=w260) -> (size(s)=w262:i32)
          n97 = Initialize Array(0.4 ("element"), w262) -> (w259:dbl[])
          n98 = call "tcpCmdArrayToZ_modify.vi"("Delay (sec)"=w259, "error in (no error)"=w256, "Timeout (ms)"=w265, "Command array"=w260, "connection ID in"=w266) -> ()  [unwired: 2 in, 5 out]
        }
        frame "Griffin" {
          w268 = string[] ["main", "Hardware Control Layer", "Beamforming", "BImage"]  # ws, mod, freq menu commands
          n99 = Format Into String(format string="IsCPAEn %d" ("Format String"), w269) -> (resulting string=w274:string)  [unwired: 2 in, 1 out]
          n100 = Build Array (concatenate)(w268, w274) -> (w271:string[])
          n101 = Array Size(array=w271) -> (size(s)=w273:i32)
          n102 = Initialize Array(0.4 ("element"), w273) -> (w270:dbl[])
          n103 = call "tcpCmdArrayToZ_modify.vi"("Delay (sec)"=w270, "error in (no error)"=w267, "Timeout (ms)"=w276, "Command array"=w271, "connection ID in"=w277) -> ()  [unwired: 2 in, 5 out]
        }
        frame Default {
        }
      }
    }
    frame #8 {
      n104 = global read "Thermal_type.vi" "System \nSelection"() -> (w282:enum32{"Common", "Frosk", "Griffin", "K2"})
      n105 = case shown="\"Griffin\"" w282 {
        tunnel: [0.0 w287 w300] -> w278
        tunnel: w281 -> [_ w286 w299]
        tunnel: w280 -> [_ w285 w298]
        tunnel: w279 -> [_ w284 w297]
        frame "Common", Default {
        }
        frame "Griffin" {
          w288 = string[] ["main", "Hardware Control Layer", "Beamforming", "BImage", "IsCPAEn"]  # ws, mod, freq menu commands
          n106 = Array Size(array=w288) -> (size(s)=w293:i32)
          n107 = Initialize Array(0.0 ("원소"), w293) -> (w295:dbl[])
          n108 = call "tcpCmdArrayToZ_modify.vi"("Delay (sec)"=w295, "error in (no error)"=w284, "Timeout (ms)"=w285, "Command array"=w288, "connection ID in"=w286) -> ("Receive array"=w294:string[])  [unwired: 2 in, 4 out]
          n109 = Decrement(x=w293) -> (x-1=w291:i32)
          n110 = Index Array(array=w294, index=w291) -> (element=w292:string)
          n111 = Match Pattern(string=w292, regular expression="250 " ("정규식")) -> (after substring=w290:string)  [unwired: 1 in, 3 out]
          n112 = Fract/Exp String To Number(string=w290) -> (number=w287:dbl)  [unwired: 3 in, 1 out]
        }
        frame "K2" {
          w301 = string[] ["main", "Hardware Control Layer", "Fe", "BImage", "IsCPAEn"]  # ws, mod, freq menu commands
          n113 = Array Size(array=w301) -> (size(s)=w306:i32)
          n114 = Initialize Array(0.0 ("원소"), w306) -> (w308:dbl[])
          n115 = call "tcpCmdArrayToZ_modify.vi"("Delay (sec)"=w308, "error in (no error)"=w297, "Timeout (ms)"=w298, "Command array"=w301, "connection ID in"=w299) -> ("Receive array"=w307:string[])  [unwired: 2 in, 4 out]
          n116 = Decrement(x=w306) -> (x-1=w304:i32)
          n117 = Index Array(array=w307, index=w304) -> (element=w305:string)
          n118 = Match Pattern(string=w305, regular expression="250 " ("정규식")) -> (after substring=w303:string)  [unwired: 1 in, 3 out]
          n119 = Fract/Exp String To Number(string=w303) -> (number=w300:dbl)  [unwired: 3 in, 1 out]
        }
      }
    }
    frame #9 {
      n120 = call "Command_verification_SA test.vi"("time out"=w334, "connection ID"=w335) -> ("Get_mea_condition"=w317:T4, "RLE data"=w313:string)  [unwired: 1 in]
      n121 = Unbundle By Name(w316) -> ("TxPulseRleA"=w314:string, "IsCPAEn"=w311:i16)
      n122 = Unbundle By Name(w336) -> ("isTxAperModulationEn"=w333:i16, "txpgWaveformStyle"=w315:i16, "numTxCycles"=w332:dbl, "numTxElements"=w331:i16)
      n123 = Unbundle By Name(w317) -> ("isTxAperModulationEn"=w330:i16, "txpgWaveformStyle"=w329:i16, "txFrequencyIndex"=w328:i32, "RoiLateralSpan"=w327:dbl, "RoiLateralMin"=w326:dbl, "numTxCycles"=w325:dbl, "numTxElements"=w324:i16)
      n124 = Build Array(w330, w329, w328, w327, w326, w325, w324, w310) -> (w323:dbl[])
      n125 = Build Array(w333, w315, w340, w339, w338, w332, w331, w311) -> (w322:dbl[])
      n126 = Equal?(x=w322, y=w323) -> (x = y?=w319:bool[])
      "All_param_veri" <- w319
      n127 = case shown="0" w315 {
        tunnel: w314 -> [_ w344]
        tunnel: w313 -> [_ w343]
        tunnel: [TRUE w342] -> w312
        frame Default {
        }
        frame 0 {
          n128 = Equal?(x=w344, y=w343) -> (x = y?=w342:bool)
        }
      }
      n129 = Array Size(array=w319) -> (size(s)=w318:i32)
      n130 = Boolean To (0,1)(Boolean=w319) -> (0, 1=w321:i16[])
      n131 = Add Array Elements(numeric array=w321) -> (sum=w320:i16)
      "Pass_count" <- w320
      n132 = Equal?(x=w320, y=w318) -> (x = y?=w337:bool)
      "veri_P/F" <- w337
      "meas_temparature_Output" <- w336
    }
    frame #10 {
      w357 = 100.0
      # "Set voltage and volt supply channel"
      n133 = Unbundle By Name(w354) -> ("VTxIndex"=w350:i8, "SysPulserSelA"=w345:i16)
      n134 = Unbundle By Name(w359) -> ("pulseVoltage"=w355:dbl)
      n135 = Multiply(x=w357, y=w355) -> (x*y=w358:dbl)
      n136 = Round To Nearest(number=w358) -> (nearest integer value=w356:dbl)
      n137 = Divide(x=w356, y=w357) -> (x/y=w348:dbl)
      n138 = global read "Thermal_type.vi" "System \nSelection"() -> (w353:enum32{"Common", "Frosk", "Griffin", "K2"})
      n139 = case shown="\"Griffin\"" w353 {
        tunnel: [w365 w374 w384] -> w347
        tunnel: w348 -> [w364 w378 w388]
        tunnel: w350 -> [_ w379 w389]
        tunnel: w352 -> [w363 w383 w394]
        tunnel: w351 -> [w362 w376 w386]
        tunnel: w349 -> [w361 w382 w393]
        tunnel: [TRUE ("x = y?") w375 w385] -> w346
        tunnel: w345 -> [_ _ w391]
        frame "Common", "Frosk", Default {
          w372 = string[] ["main", "Hardware Control Layer", "Beamforming", "Common"]  # Voltage menu commands
          n140 = Format Into String(format string="PulseVoltageA poke %d %.2f" ("Format String"), i8 0 ("입력 1"), w364) -> (resulting string=w371:string)  [unwired: 2 in, 1 out]
          n141 = Build Array (concatenate)(w372, w371) -> (w367:string[])
          n142 = Array Size(array=w367) -> (size(s)=w370:i32)
          n143 = Initialize Array(0.4 ("element"), w370) -> (w368:dbl[])
          n144 = call "tcpCmdArrayToZ_modify.vi"("Delay (sec)"=w368, "error in (no error)"=w361, "Timeout (ms)"=w362, "Command array"=w367, "connection ID in"=w363) -> ("error out"=w365:errorcluster)  [unwired: 2 in, 4 out]
        }
        frame "Griffin" {
          n145 = call "VTx_control_Juniper.vi"("VTx_Voltage"=w378, "VTxIndex_In"=w379, "error in (no error)"=w382, "VTx1_voltage"=93.0, "Timeout (ms)"=w376, "connection ID in"=w383) -> ("error out"=w377:errorcluster, "connection ID out"=w380:refnum<k5>)  [unwired: 4 in]
          n146 = call "Control_verify_voltage.vi"("Timeout (ms)"=w376, "에러 입력(에러 없음)"=w377, "VTx_Voltage"=w378, "VTxIndex_In"=w379, "TCP 네트워크 연결 입력"=w380) -> ("에러 출력"=w374:errorcluster, "Verify_voltage"=w375:bool)  [unwired: 2 in, 3 out]
        }
        frame "K2" {
          n147 = call "VTx_control_K2.vi"("VTx_Voltage"=w388, "VTxIndex_In"=w389, "SystemPulerSelA"=w391, "error in (no error)"=w393, "CW/SCW"=FALSE, "Timeout (ms)"=w386, "connection ID in"=w394) -> ("error out"=w387:errorcluster, "connection ID out"=w390:refnum<k5>)  [unwired: 3 in]
          n148 = call "Control_verify_voltage.vi"("Timeout (ms)"=w386, "에러 입력(에러 없음)"=w387, "VTx_Voltage"=w388, "VTxIndex_In"=w389, "TCP 네트워크 연결 입력"=w390) -> ("에러 출력"=w384:errorcluster, "Verify_voltage"=w385:bool)  [unwired: 2 in, 3 out]
        }
      }
      "error out" <- w347
    }
    frame #11 {
      n149 = Compound Arithmetic op=AND(w395, w398, w397) -> (w396:bool)
      n150 = case shown="거짓" w396 {
        tunnel: w400 -> [w402 _]
        tunnel: w399 -> [w401 _]
        frame False {
          n151 = stacked-sequence {
            tunnel: w402 -> [w404 _]
            tunnel: w401 -> [w403 _]
            frame #0 {
              # "Close telnet connection, write log"
              # "write \"quit\" even\nif error exists"
              n152 = TCP Write(connection ID=w404, data in="quit\n", 9:w403) -> (connection ID out=w408:refnum<k5>, error out=w406:errorcluster)  [unwired: 1 in, 1 out]
              n153 = TCP Close Connection(connection ID=w408, error in (no error)=w406) -> (error out=→"error out 2":errorcluster)  [unwired: 1 in, 1 out]
            }
            frame #1 {
              n154 = One Button Dialog(message="Parameters are Not matched" ("메시지"), button name ("OK")="Stop" ("버튼 이름(\"확인\")")) -> (true=w410:bool)
              n155 = Stop(stop? (T)=w410) -> ()
            }
          }
        }
        frame True {
        }
      }
    }
    frame #12 {
      n156 = global read "Thermal_type.vi" "Measurement Type"() -> (w412:enum32{"Volt", "SA"})
      n157 = call "Monitoring PRF.vi"("Measurement Type"=w412, "timeout (ms)"=w413, "TCP from Orchid in"=w414) -> ("PRF"=→"Actual PRF":dbl)  [unwired: 6 in, 1 out]
    }
  }
